vi "cleanQueue.vi"(2 "String":string, 3 "queue in":refnum<queue>) -> (1 "queue in":refnum<queue>)   [LabVIEW 2013]
doc: "Checks the queue to see if the program should terminate. If not, and string is empty deletes the first element. If string is not empty, flushes queue and enqueues an empty string and then string."
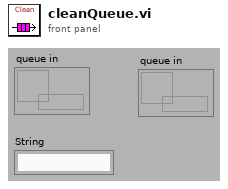
[diagram p1: front panel]
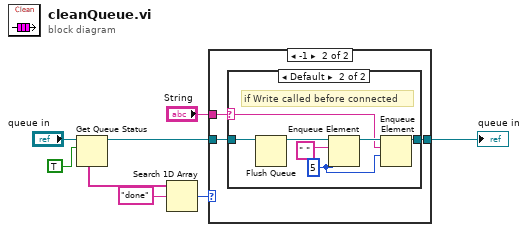
[diagram p0: block diagram]
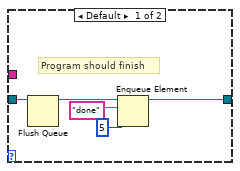
[diagram p2: hidden frame]
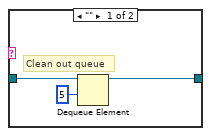
[diagram p3: hidden frame]
diagram:
  n1 = Get Queue Status(queue="queue in", return elements? (F)=TRUE) -> (queue out=w7:refnum<queue>, elements=w3:string[])  [unwired: 1 in, 6 out]
  n2 = Search 1D Array(1D array=w3, element="done") -> (index of element=w6:i32)  [unwired: 1 in]
  n3 = case shown="-1" w6 {
    tunnel: w7 -> [w13 w16]
    tunnel: "String" -> [_ w15]
    tunnel: [w10 w14] -> w1
    frame Default {
      # "Program should finish"
      n4 = Flush Queue(queue=w13) -> (queue out=w12:refnum<queue>)  [unwired: 1 in, 2 out]
      n5 = Enqueue Element(queue=w12, element="done", timeout in ms (-1)=5) -> (queue out=w10:refnum<queue>)  [unwired: 1 in, 2 out]
    }
    frame -1 {
      n6 = case shown="Default" w15 {
        selector: w15 -> [_ w20]
        tunnel: w16 -> [w19 w25]
        tunnel: [w18 w22] -> w14
        frame "" {
          # "Clean out queue"
          n7 = Dequeue Element(queue=w19, timeout in ms (-1)=5) -> (queue out=w18:refnum<queue>)  [unwired: 1 in, 3 out]
        }
        frame Default {
          w21 = 5 ("timeout in ms (-1)")
          # "if Write called before connected"
          n8 = Flush Queue(queue=w25) -> (queue out=w24:refnum<queue>)  [unwired: 1 in, 2 out]
          n9 = Enqueue Element(queue=w24, element=" ", timeout in ms (-1)=w21) -> (queue out=w26:refnum<queue>)  [unwired: 1 in, 2 out]
          n10 = Enqueue Element(queue=w26, element=w20, timeout in ms (-1)=w21) -> (queue out=w22:refnum<queue>)  [unwired: 1 in, 2 out]
        }
      }
    }
  }
  "queue in" <- w1
